vi "Write TC Parameters.vi"(4 "Error In":errorcluster, 6 "TC Parameters":T1, 7 "Set TC Parameters in":refnum<class "Remote Access Commands_Set TC Parameters.lvclass">) -> (0 "Error Out":errorcluster, 3 "Set TC Parameters out":refnum<class "Remote Access Commands_Set TC Parameters.lvclass">)   [LabVIEW 2015, in "Startup Processes.lvlib" / "Remote Access Commands_Set TC Parameters.lvclass"]
uses:
  Remote Access Commands_Set TC Parameters.lvclass
  _typedefs/TC Setup Parameters.ctl
  Remote Access Commands_Set TC Parameters.lvclass/Remote Access Commands_Set TC Parameters.ctl
  Startup Processes.lvlib
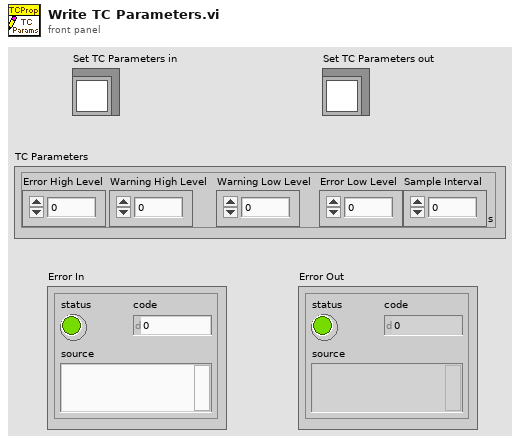
[diagram p1: front panel]
types:
  T1 = typedef "Startup Processes.lvlib/TC Setup Parameters.ctl" = cluster{"Error High Level":dbl, "Warning High Level":dbl, "Warning Low Level":dbl, "Error Low Level":dbl, "Sample Interval":dbl[unit]}
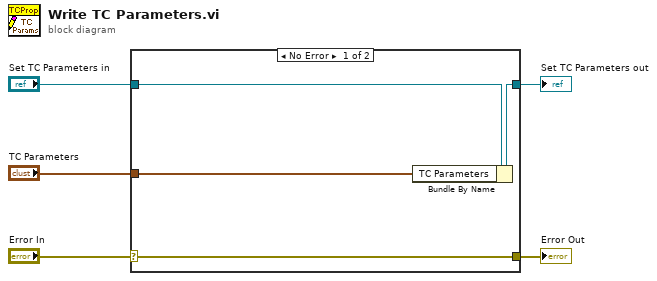
[diagram p0: block diagram]
diagram:
  n1 = case shown="No Error" "Error In" {
    selector: "Error In" -> [w9 w10]
    tunnel: [w9 w10] -> w4
    tunnel: [w7 w11] -> w2
    tunnel: "Set TC Parameters in" -> [w8 w11]
    tunnel: "TC Parameters" -> [w6 _]
    frame No Error {
      n2 = Bundle By Name(cluster=w8, "TC Parameters"=w6) -> (w7:refnum<class "Remote Access Commands_Set TC Parameters.lvclass">)
    }
    frame Error {
    }
  }
  "Error Out" <- w4
  "Set TC Parameters out" <- w2
